vi "CreateHandleHolder.vi"(7 "Min Level":T1, 10 "Handle":refnum<class "LoggingHandle.lvclass">, 11 "Name":string) -> (3 "HandleHolder out":refnum<class "HandleHolder.lvclass">)   [LabVIEW 2024, in "HandleHolder.lvclass"]
uses:
  HandleHolder.lvclass
  Shared/Level.ctl
  LogHandle/Interface/LoggingHandle.lvclass
  HandleHolder.lvclass/HandleHolder.ctl
  Shared/LoggerShared.lvlib
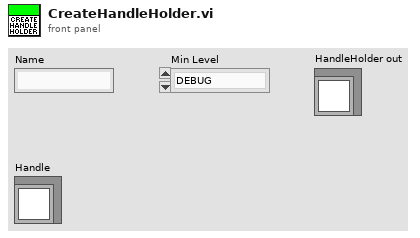
[diagram p1: front panel]
types:
  T1 = typedef "LoggerShared.lvlib/Level.ctl" = enum16{"DEBUG", "INFO", "WARNING", "ERROR", "CRITICAL"}
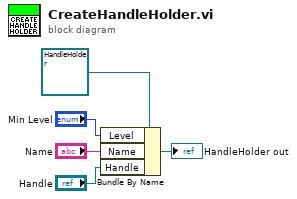
[diagram p0: block diagram]
diagram:
  n1 = Bundle By Name(cluster=refnum<class "HandleHolder.lvclass"> refnum ("HandleHolder in"), "Level"="Min Level", "Name"="Name", "Handle"="Handle") -> (→"HandleHolder out":refnum<class "HandleHolder.lvclass">)
